vi "ARMS_5.vi"() -> ()   [LabVIEW 2018]
uses:
  <vilib>/Analysis/Matrix/Datatypes/RealMatrix.ctl
  <vilib>/Analysis/Matrix/NI_Matrix.lvlib
panel:
  out "3D Picture 2":refnum<vi>(3d-picture)
  out "Array 2":dbl[](array[numeric])
  out "A x B 3":T1=[[1.0, 0.0, 0.0, 0.0], [0.0, 6.123233995736766e-17, 1.0, 0.0], [0.0, -1.0, 6.123233995736766e-17, 0.0], [0.0, 0.0, 0.0, 1.0]] format="%#_2g"
  in  "Phi":dbl(slide) scale=90.0..-90.0
  out "Array":dbl[](array[numeric])
  in  "stop":bool
  out "A x B 2":T1=[[1.0, 0.0, 0.0, 0.0], [0.0, 6.123233995736766e-17, 1.0, 0.0], [0.0, -1.0, 6.123233995736766e-17, 0.0], [0.0, 0.0, 0.0, 1.0]] format="%#_2g"
  out "3D Picture 3":refnum<vi>(3d-picture)
  in  "X":dbl(slide) scale=0.0..2.0
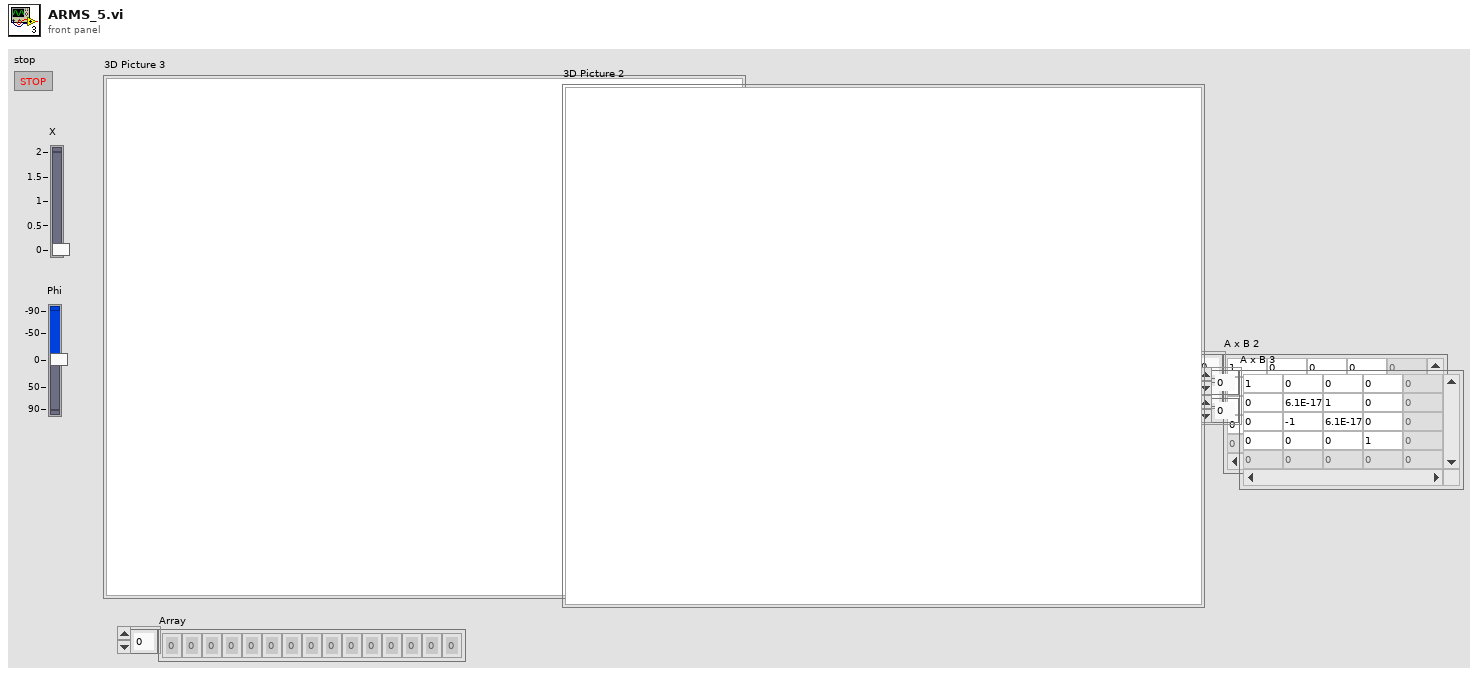
[diagram p1: front panel]
types:
  T1 = typedef "NI_Matrix.lvlib/RealMatrix.ctl" = dbl[][]
  T2 = cluster{"Theta":dbl, "d":dbl, "a":dbl, "alpha (degrees)":dbl}[]
  T3 = cluster{"Theta":dbl, "d":dbl, "a":dbl, "alpha (degrees)":dbl}
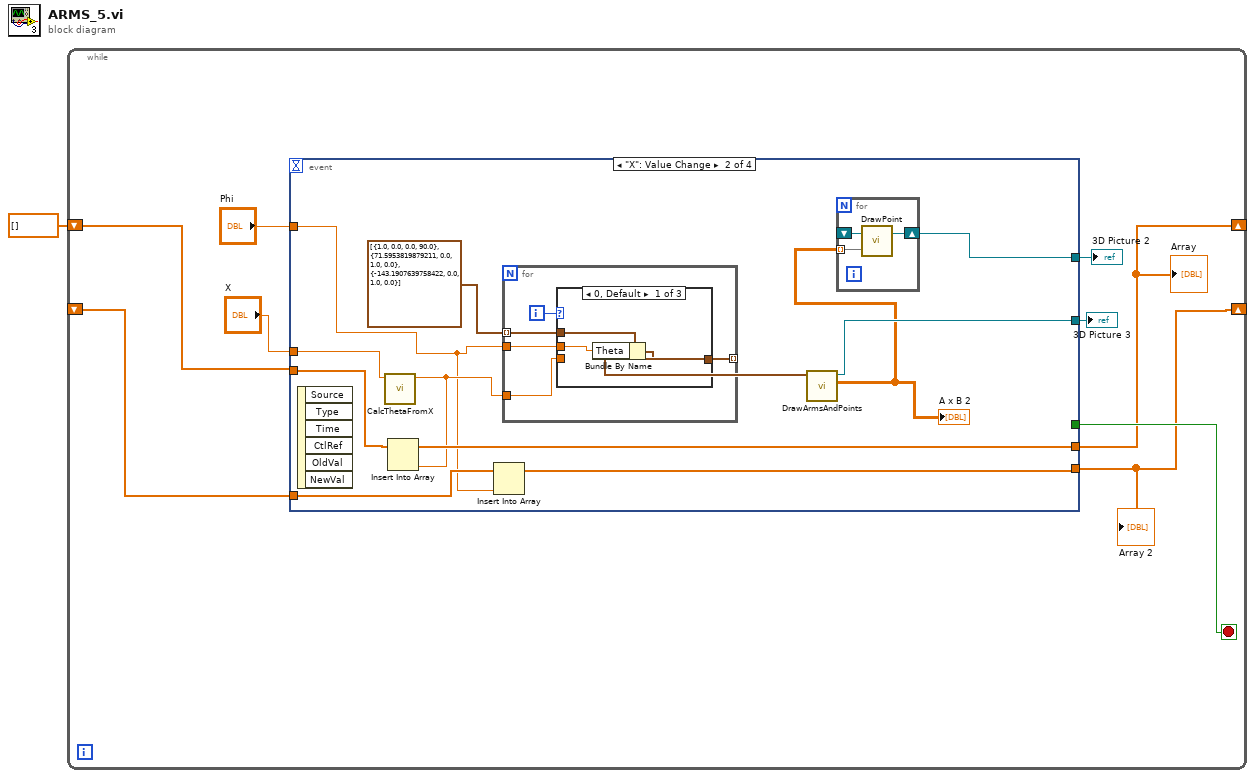
[diagram p0: block diagram]
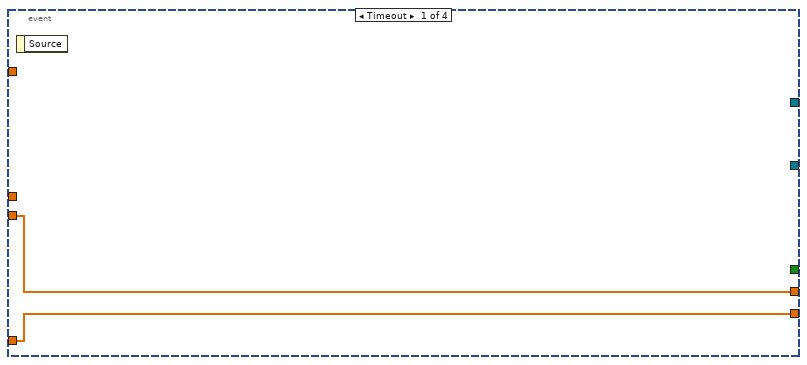
[diagram p2: hidden frame]
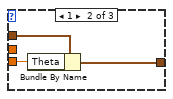
[diagram p3: hidden frame]
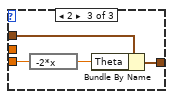
[diagram p4: hidden frame]
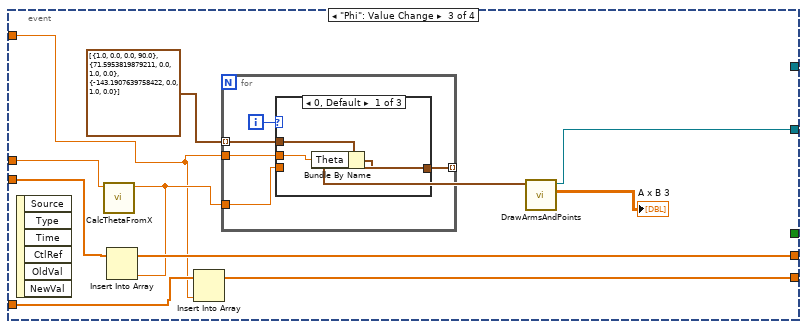
[diagram p5: hidden frame]
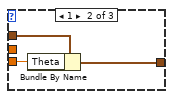
[diagram p6: hidden frame]
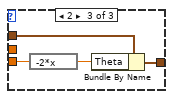
[diagram p7: hidden frame]
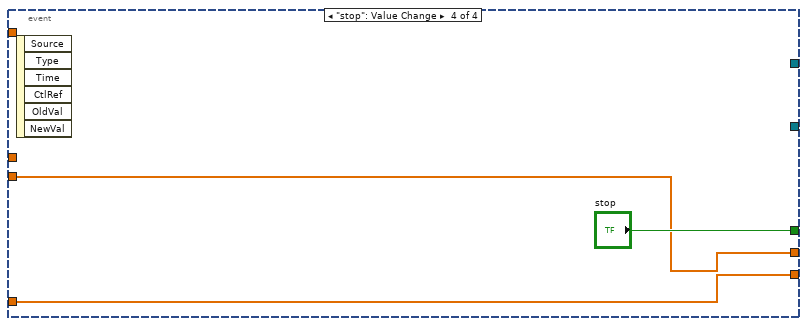
[diagram p8: hidden frame]
diagram:
  n1 = while {
    shift-right: [w6] -> _
    shift-left: dbl[] [] -> [w7]
    shift-right: [w3] -> _
    shift-left: _ -> [w4]
    stop <- w8 stop-if-true
    n2 = event shown="[1] \"X\": Value Change" {
      selector: _ -> [_ _ _ _]
      dyn-events: _ -> [_ _ _ _]
      timeout: _ -> [_ _ _ _]
      tunnel: "X" -> [_ w24 w53 _]
      tunnel: [_ w21 w50 _] -> w9
      tunnel: [_ _ _ "stop"] -> w8
      tunnel: [w12 w19 w47 w70] -> w6
      tunnel: w7 -> [w12 w20 w48 w70]
      tunnel: "Phi" -> [_ w16 w44 _]
      tunnel: w4 -> [w11 w17 w45 w69]
      tunnel: [w11 w15 w43 w69] -> w3
      tunnel: [_ w14 _ _] -> w2
      event Timeout {
        n3 = event-data() -> ()  [unwired: 1 in, 1 out]
      }
      event "X": Value Change {
        n4 = event-data() -> ()  [unwired: 1 in, 6 out]
        n5 = call "CalcThetaFromX.vi"("X"=w24) -> ("Numeric"=w18:dbl)  [unwired: 10 in]
        n6 = Insert Into Array(array=w20, new element=w18) -> (w19:dbl[])  [unwired: 1 in]
        n7 = Insert Into Array(array=w17, new element=w16) -> (w15:dbl[])  [unwired: 1 in]
        n8 = for {
          tunnel: w18 -> [w31]
          tunnel: T2 [{"Theta"=1.0, "d"=0.0, "a"=0.0, "alpha (degrees)"=90.0}, {"Theta"=71.5953819879211, "d"=0.0, "a"=1.0, "alpha (degrees)"=0.0}, {"Theta"=-143.1907639758422, "d"=0.0, "a"=1.0, "alpha (degrees)"=0.0}] ("Joints") -> [w30] mode=indexing
          tunnel: [w29] -> w22 mode=indexing
          tunnel: w16 -> [w28]
          i -> [w32]
          n9 = case shown="0, Default" w32 {
            tunnel: w31 -> [_ w37 w41]
            tunnel: w30 -> [w35 w38 w42]
            tunnel: [w33 w36 w40] -> w29
            tunnel: w28 -> [w34 _ _]
            frame 0, Default {
              n10 = Bundle By Name(cluster=w35, "Theta"=w34) -> (w33:T3)
            }
            frame 1 {
              n11 = Bundle By Name(cluster=w38, "Theta"=w37) -> (w36:T3)
            }
            frame 2 {
              n12 = expression code="-2*x"(w41) -> (w39:dbl)
              n13 = Bundle By Name(cluster=w42, "Theta"=w39) -> (w40:T3)
            }
          }
        }
        n14 = call "DrawArmsAndPoints.vi"("Array"=w22) -> ("A x B"=w13:T1, "SceneObject out"=w21:refnum<vi>)  [unwired: 9 in]
        "A x B 2" <- w13
        n15 = for {
          shift-right: [w26] -> w14
          shift-left: _ -> [w27]
          tunnel: w13 -> [w25] mode=indexing
          n16 = call "DrawPoint.vi"("Start"=w25, "Stage in"=w27) -> ("Stage out"=w26:refnum<vi>)  [unwired: 1 in]
        }
      }
      event "Phi": Value Change {
        n17 = event-data() -> ()  [unwired: 1 in, 6 out]
        n18 = call "CalcThetaFromX.vi"("X"=w53) -> ("Numeric"=w46:dbl)  [unwired: 10 in]
        n19 = Insert Into Array(array=w48, new element=w46) -> (w47:dbl[])  [unwired: 1 in]
        n20 = Insert Into Array(array=w45, new element=w44) -> (w43:dbl[])  [unwired: 1 in]
        n21 = for {
          tunnel: w46 -> [w57]
          tunnel: T2 [{"Theta"=1.0, "d"=0.0, "a"=0.0, "alpha (degrees)"=90.0}, {"Theta"=71.5953819879211, "d"=0.0, "a"=1.0, "alpha (degrees)"=0.0}, {"Theta"=-143.1907639758422, "d"=0.0, "a"=1.0, "alpha (degrees)"=0.0}] ("Joints") -> [w56] mode=indexing
          tunnel: [w55] -> w51 mode=indexing
          tunnel: w44 -> [w54]
          i -> [w58]
          n22 = case shown="0, Default" w58 {
            tunnel: w57 -> [_ w63 w67]
            tunnel: w56 -> [w61 w64 w68]
            tunnel: [w59 w62 w66] -> w55
            tunnel: w54 -> [w60 _ _]
            frame 0, Default {
              n23 = Bundle By Name(cluster=w61, "Theta"=w60) -> (w59:T3)
            }
            frame 1 {
              n24 = Bundle By Name(cluster=w64, "Theta"=w63) -> (w62:T3)
            }
            frame 2 {
              n25 = expression code="-2*x"(w67) -> (w65:dbl)
              n26 = Bundle By Name(cluster=w68, "Theta"=w65) -> (w66:T3)
            }
          }
        }
        n27 = call "DrawArmsAndPoints.vi"("Array"=w51) -> ("A x B"=→"A x B 3":T1, "SceneObject out"=w50:refnum<vi>)  [unwired: 9 in]
      }
      event "stop": Value Change {
        n28 = event-data() -> ()  [unwired: 1 in, 6 out]
      }
    }
    "3D Picture 3" <- w9
    "Array" <- w6
    "Array 2" <- w3
    "3D Picture 2" <- w2
  }
